vi "MAD_Laborator_03.vi"() -> ()   [LabVIEW 2018]
uses:
  <vilib>/DAQmx/write.llb/DAQmx Write (Analog DBL 1Chan 1Samp).vi
  <vilib>/DAQmx/read.llb/DAQmx Read (Analog 1D DBL 1Chan NSamp).vi
  <vilib>/DAQmx/miscellaneous.llb/DAQmx Fill In Error Info.vi
  <vilib>/measure/NI_MABase.lvlib
panel:
  out "Trigger":dbl[](graph)
  in  "stop 2":bool
  in  "stop":bool
  out "size(s)":i32
  out "error out":errorcluster
  in  "frequency":dbl=10.0 format="%0.2p"
  in  "square wave duty cycle (%)":dbl=50.0 format="%0.2f"
  in  "sampling info":cluster{"Fs":dbl, "#s":dbl}={"Fs"=1000.0, "#s"=1000.0} {"Fs" format="%.2p"}
  in  "signal type 2":T1(ring)
  out "generate":dbl[](graph)
  out "aquire":dbl[](graph)
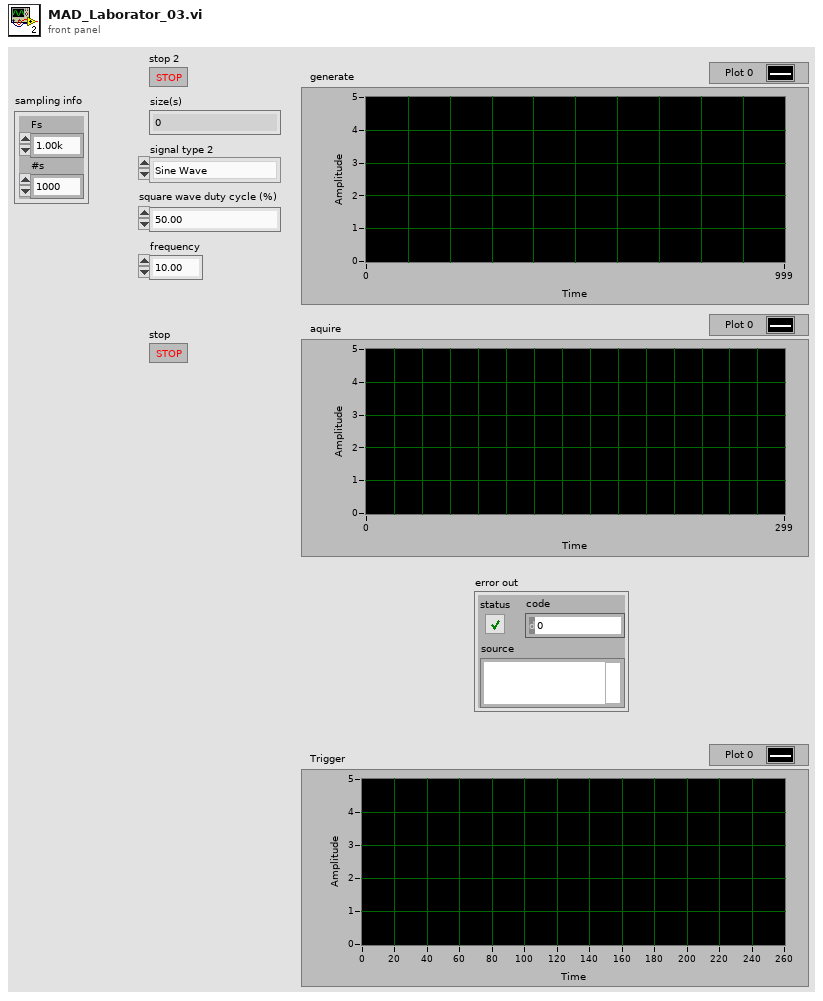
[diagram p1: front panel]
types:
  T1 = enum16{"Sine Wave", "Triangle Wave", "Square Wave", "Sawtooth Wave"}
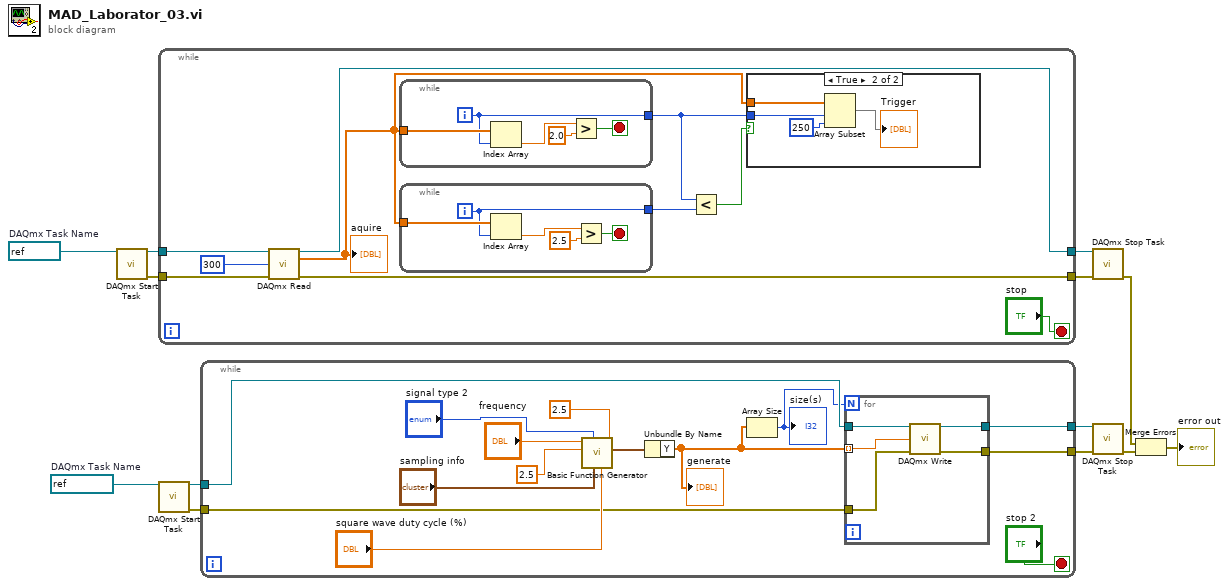
[diagram p0: block diagram]
diagram:
  w7 = refnum<k21> "V_OUT"  # DAQmx Task Name
  w12 = refnum<k21> "V_IN"  # DAQmx Task Name
  n1 = call <vilib>:"DAQmx Start Task.vi"("task/channels in"=w12) -> ("task out"=w11:refnum<k21>, "error out"=w13:errorcluster)  [unwired: 13 in]
  n2 = while {
    tunnel: w13 -> [w23]
    tunnel: w11 -> [w22]
    tunnel: [w20] -> w10
    tunnel: [w19] -> w9
    stop <- "stop" stop-if-true
    n3 = call-poly <vilib>:"DAQmx Read.vi"("task/channels in"=w22, "number of samples per channel"=300, "error in"=w23) -> ("task out"=w20:refnum<k21>, "data"=w15:dbl[], "error out"=w19:errorcluster)  [unwired: 10 in]
    "aquire" <- w15
    n4 = while {
      tunnel: w15 -> [w37]
      tunnel: [w33] -> w14
      i -> [w33]
      stop <- w34 stop-if-true
      n5 = Index Array(array=w37, index=w33) -> (element=w36:dbl)
      n6 = Greater?(x=w36, y=2.0) -> (0:w34:bool)
    }
    n7 = while {
      tunnel: w15 -> [w32]
      tunnel: [w28] -> w17
      i -> [w28]
      stop <- w29 stop-if-true
      n8 = Index Array(array=w32, index=w28) -> (element=w31:dbl)
      n9 = Greater?(x=w31, y=2.5) -> (0:w29:bool)
    }
    n10 = Less?(x=w14, y=w17) -> (x < y?=w16:bool)
    n11 = case shown="True" w16 {
      tunnel: w15 -> [_ w27]
      tunnel: w14 -> [_ w24]
      frame False {
      }
      frame True {
        n12 = Array Subset(array=w27, index=w24, length=250) -> (→"Trigger":dbl[])
      }
    }
  }
  n13 = call <vilib>:"DAQmx Start Task.vi"("task/channels in"=w7) -> ("task out"=w6:refnum<k21>, "error out"=w5:errorcluster)  [unwired: 13 in]
  n14 = while {
    tunnel: w6 -> [w44]
    tunnel: w5 -> [w43]
    tunnel: [w42] -> w4
    tunnel: [w41] -> w3
    stop <- "stop 2" stop-if-true
    n15 = call <vilib>:"Basic Function Generator.vi"("offset"=2.5, "square wave duty cycle (%)"="square wave duty cycle (%)", "sampling info"="sampling info", "signal type"="signal type 2", "amplitude"=2.5, "frequency"="frequency") -> ("signal out"=w51:waveform(dbl))  [unwired: 3 in, 2 out]
    n16 = Unbundle By Name(w51) -> ("Y"=w39:dbl[])
    "generate" <- w39
    n17 = Array Size(array=w39) -> (size(s)=w40:i32)
    "size(s)" <- w40
    n18 = for {
      N: w40 -> [_]
      tunnel: w44 -> [w56]
      tunnel: w43 -> [w55]
      tunnel: [w54] -> w42
      tunnel: [w53] -> w41
      tunnel: w39 -> [w52] mode=indexing
      n19 = call-poly <vilib>:"DAQmx Write.vi"("task/channels in"=w56, "data"=w52, "error in"=w55) -> ("task out"=w54:refnum<k21>, "error out"=w53:errorcluster)  [unwired: 10 in, 1 out]
    }
  }
  n20 = call <vilib>:"DAQmx Stop Task.vi"("task/channels in"=w10, "error in"=w9) -> ("error out"=w8:errorcluster)  [unwired: 12 in, 1 out]
  n21 = call <vilib>:"DAQmx Stop Task.vi"("task/channels in"=w4, "error in"=w3) -> ("error out"=w2:errorcluster)  [unwired: 12 in, 1 out]
  n22 = Merge Errors(w8, w2) -> (→"error out":errorcluster)
